vi "Grab Image.vi"(8 "error in":errorcluster, 11 "IMG_SRC in":refnum<class "IMG_SRC.lvclass">) -> (0 "error out":errorcluster, 3 "IMG_SRC out":refnum<class "IMG_SRC.lvclass">)   [LabVIEW 2018, in "IMG_SRC.lvlib" / "IMG_SRC.lvclass"]
uses:
  IMG_SRC.lvclass
  IMG_SRC.lvclass/IMG_SRC.ctl
  builds/Camera.lvlibp/Camera.lvclass
  C:/Users/Ron.Dexter.LUMINARTECH/Desktop/builds/Camera.lvlibp/Camera.lvclass
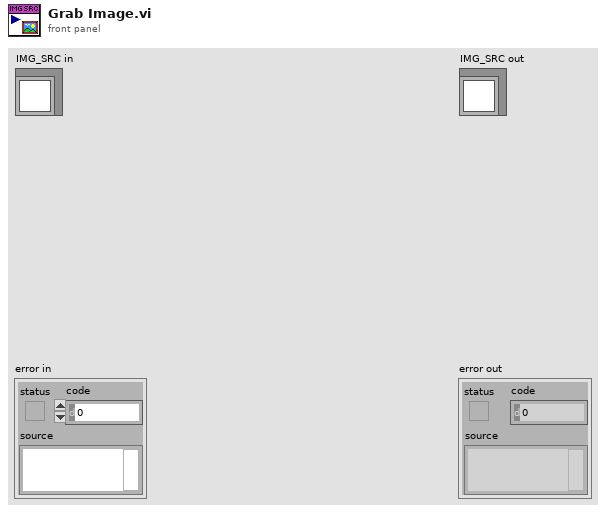
[diagram p1: front panel]
types:
  T1 = typedef "IMAQ Image.ctl" = refnum<image>
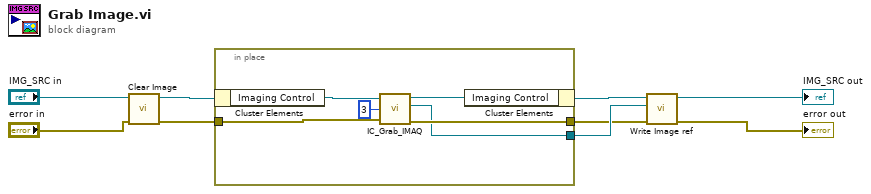
[diagram p0: block diagram]
diagram:
  n1 = call "Clear Image.vi"("error in"="error in", "IMG_SRC in"="IMG_SRC in") -> ("error out"=w6:errorcluster, "IMG_SRC out"=w8:refnum<class "IMG_SRC.lvclass">)  [unwired: 8 in]
  n2 = in-place {
    in-place-border: [w13] -> w3
    in-place-border: w6 -> [w12]
    in-place-border: [w10] -> w4
    n3 = in-place-cluster #1(w8) -> ("Imaging Control"=w15:refnum<k7>)
    n4 = call <userlib>:"IC_Grab_IMAQ.vi"("ICImagingControl In"=w15, "BorderSize"=3, "Error In (no error)"=w12) -> ("ICImagingControl Out"=w14:refnum<k7>, "Image Out"=w10:T1, "Error Out"=w13:errorcluster)  [unwired: 1 out]
    n5 = in-place-cluster #1("Imaging Control"=w14) -> (w5:refnum<class "IMG_SRC.lvclass">)
  }
  n6 = call "Write Image ref.vi"("error in (no error)"=w3, "Image"=w4, "Camera in"=w5) -> ("error out"=→"error out":errorcluster, "Camera out"=→"IMG_SRC out":refnum<class "IMG_SRC.lvclass">)  [unwired: 7 in]
